vi "EnableDisable - Right Click.vi"(8 "error in (no error)":errorcluster, 11 "Node Ptr":u64 format="%.0x") -> (0 "error out":errorcluster)   [LabVIEW 2013, in "AIT 664 Custom Device.lvlib"]
uses:
  AIT 664 Custom Device.lvlib
  Controls and Global/Global.vi
  <vilib>/NI Veristand/Custom Device API/Custom Device API.lvlib
panel:
  in  "Tag":string
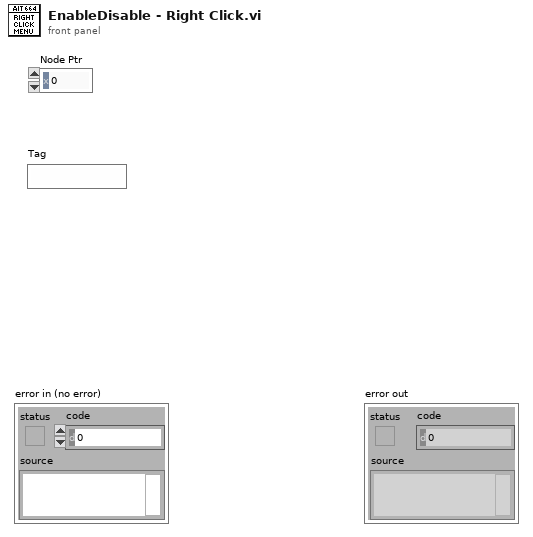
[diagram p1: front panel]
types:
  T1 = typedef "Custom Device API.lvlib/Custom Device Item Ref.ctl" = u64
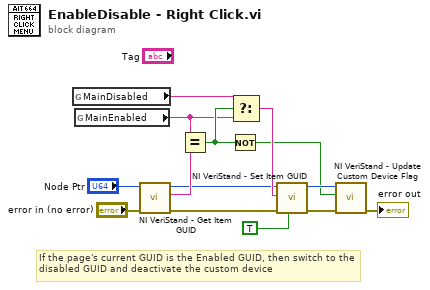
[diagram p0: block diagram]
diagram:
  # "If the page's current GUID is the Enabled GUID, then switch to the disabled GUID and deactivate the custom device"
  n1 = global read "Global.vi" "MainDisabled"() -> (w2:string)
  n2 = global read "Global.vi" "MainEnabled"() -> (w3:string)
  n3 = call <vilib>:"NI VeriStand - Get Item GUID.vi"("error in (no error)"="error in (no error)", "Item Ref in"="Node Ptr") -> ("error out"=w12:errorcluster, "GUID"=w14:string, "Item Ref out"=w1:T1)  [unwired: 7 in]
  n4 = Equal?(x=w3, y=w14) -> (x = y?=w8:bool)
  n5 = Not(x=w8) -> (.not. x?=w7:bool)
  n6 = Select(t=w2, s=w8, f=w3) -> (s? t:f=w11:string)
  n7 = call <vilib>:"NI VeriStand - Set Item GUID.vi"("Refresh System Explorer Tree? (F)"=TRUE, "error in (no error)"=w12, "GUID"=w11, "Item Ref in"=w1) -> ("error out"=w10:errorcluster, "Item Ref out"=w9:T1)  [unwired: 6 in]
  n8 = call <vilib>:"NI VeriStand - Update Custom Device Flag.vi"("error in (no error)"=w10, "Is Custom Device Active?"=w7, "Device Ref in"=w9) -> ("error out"=→"error out":errorcluster)  [unwired: 7 in, 1 out]
